vi "Ensure All Modules Exit.vi"(8 "Error in":errorcluster caption="Error in (no error)") -> (0 "Error out":errorcluster)   [LabVIEW 2017, in "CSM-Testcase.lvlib"]
uses:
  CSM-Testcase.lvlib
  src/user.lib/_NEVSTOP/Communicable State Machine(CSM)/_Support/Typedef/_CSM_List Module Scope.ctl
  src/user.lib/_NEVSTOP/Communicable State Machine(CSM)/Communicable State Machine.lvlib
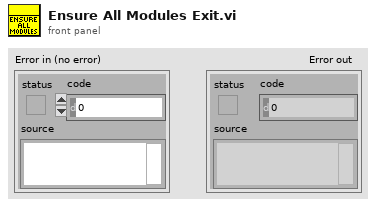
[diagram p1: front panel]
types:
  T1 = typedef "Communicable State Machine.lvlib/_CSM_List Module Scope.ctl" = enum16{"Normal", "System Only", "All"}
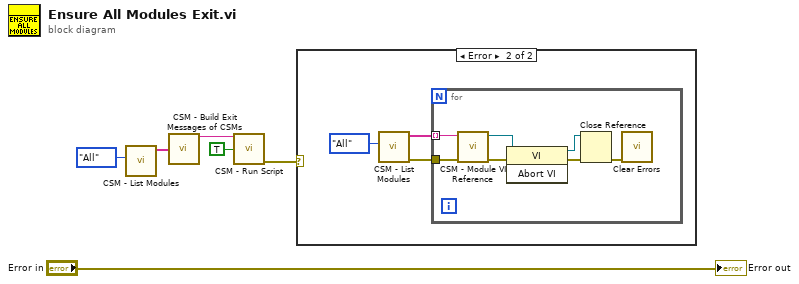
[diagram p0: block diagram]
diagram:
  n1 = call "CSM - List Modules.vi"("Scope (Normal)"=_CSM_List_Module_Scope."All") -> ("Module Names"=w3:string[])  [unwired: 9 in, 1 out]
  n2 = call "CSM - Build Exit Messages of CSMs.vi"("CSMs"=w3) -> ("States"=w5:string)  [unwired: 14 in]
  n3 = call "CSM - Run Script.vi"("CSM Scripts"=w5, "Continue If Error? (F)"=TRUE ("Continue If Error?(F)")) -> ("error out"=w1:errorcluster)  [unwired: 11 in, 2 out]
  n4 = case shown="Error" w1 {
    frame No Error {
    }
    frame Error {
      n5 = call "CSM - List Modules.vi"("Scope (Normal)"=_CSM_List_Module_Scope."All") -> ("error out"=w8:errorcluster, "Module Names"=w7:string[])  [unwired: 9 in]
      n6 = for {
        tunnel: w8 -> [w16]
        tunnel: w7 -> [w15] mode=indexing
        n7 = call "CSM - Module VI Reference.vi"("error in (no error)"=w16, "CSM Name"=w15) -> ("error out"=w13:errorcluster, "CSM Module VIRef"=w14:refnum<vi>)  [unwired: 8 in]
        n8 = invoke class="VI" method="Abort VI"(reference=w14, error in=w13) -> (reference out=w11:refnum<vi>, error out=w12:errorcluster)  [unwired: 1 in, 1 out]
        n9 = Close Reference(reference=w11, error in (no error)=w12) -> (error out=w10:errorcluster)
        n10 = call <vilib>:"Clear Errors.vi"("error in (no error)"=w10) -> ()  [unwired: 5 in, 2 out]
      }
    }
  }
  "Error out" <- "Error in"
